vi "Inc (Core).vi"(6 "Labels":map{string, string}(c390), 8 "error in (no error)":errorcluster, 10 "Step":dbl=1.0, 11 "Counter in":refnum<class "Counter.lvclass">) -> (0 "error out":errorcluster, 3 "Counter out":refnum<class "Counter.lvclass">)   [LabVIEW 2020]
uses:
  Counter.lvclass
  C:/Github-locals/PromVIEW/src/metrics/metric/Metric.lvclass
  metric/Metric.lvclass/Metric.ctl
  sample/Sample.lvclass/Sample.ctl
  sample/Read Value.vi
  sample/Write Value.vi
  sample/Write Labels.vi
  metric/Read Samples.vi
  metric/Read Name.vi
  metric/Write Samples.vi
  <vilib>/Utility/error.llb/Error Cluster From Error Code.vi
  <vilib>/ErrorRing/Error Ring.xnode
  sample/Sample.lvclass
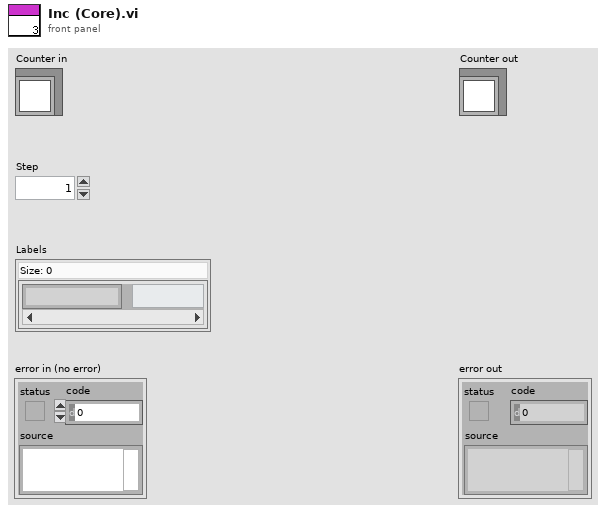
[diagram p1: front panel]
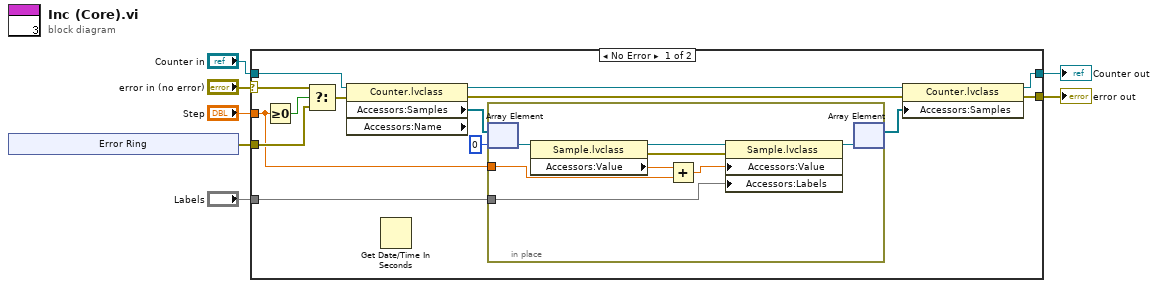
[diagram p0: block diagram]
diagram:
  n1 = xnode "Error Ring"() -> ("error out"=w1:errorcluster)
  n2 = case shown="No Error" "error in (no error)" {
    selector: "error in (no error)" -> [w19 w31]
    tunnel: [w12 w31] -> w6
    tunnel: [w13 w30] -> w4
    tunnel: "Counter in" -> [w21 w30]
    tunnel: "Step" -> [w9 _]
    tunnel: "Labels" -> [w8 _]
    tunnel: w1 -> [w18 _]
    frame No Error {
      n3 = Greater Or Equal To 0?(x=w9) -> (x >= 0?=w20:bool)
      n4 = Select(t=w19, s=w20, f=w18) -> (s? t:f=w10:errorcluster)
      n5 = property class="Counter.lvclass" props=["Accessors:Samples", "Accessors:Name"](reference=w21, error in=w10) -> (reference out=w15:refnum<class "Counter.lvclass">, error out=w11:errorcluster, "Accessors:Samples"=w17:refnum<class "Sample.lvclass">[])  [unwired: 1 out]
      n6 = Get Date/Time In Seconds() -> ()  [unwired: 1 out]
      n7 = in-place {
        in-place-border: w8 -> [w23]
        in-place-border: w9 -> [w25]
        n8 = in-place-array #1(w17, 0) -> (w29:refnum<class "Sample.lvclass">)
        n9 = property class="Sample.lvclass"(reference=w29) -> (reference out=w28:refnum<class "Sample.lvclass">, error out=w27:errorcluster, "Accessors:Value"=w26:dbl)  [unwired: 1 in]
        n10 = Add(x=w26, y=w25) -> (x+y=w24:dbl)
        n11 = property class="Sample.lvclass"(reference=w28, error in=w27, "Accessors:Value"=w24, "Accessors:Labels"=w23) -> (reference out=w22:refnum<class "Sample.lvclass">)  [unwired: 1 out]
        n12 = in-place-array #1(w22) -> (w14:refnum<class "Sample.lvclass">[])  [unwired: 1 out]
      }
      n13 = property class="Counter.lvclass"(reference=w15, error in=w11, "Accessors:Samples"=w14) -> (reference out=w13:refnum<class "Counter.lvclass">, error out=w12:errorcluster)
    }
    frame Error {
    }
  }
  "error out" <- w6
  "Counter out" <- w4
